vi "Get Custom Device Reference.vi"(8 "error in (no error)":errorcluster, 11 "Item Ref in":T1 format="%.0x") -> (0 "error out":errorcluster, 2 "Custom Device Ref":T1 format="%.0x", 3 "Item Ref out":T1 format="%.0x")   [LabVIEW 2020, in "Engine Simulation Toolkit System Explorer.lvlib"]
uses:
  Engine Simulation Toolkit System Explorer.lvlib
  <vilib>/NI VeriStand/Custom Device API/Custom Device Item Ref.ctl
  <vilib>/NI VeriStand/Custom Device Tools/Custom Device Utility Library/Search Direction.ctl
  Shared/Constants and GUIDs.vi
  <vilib>/NI VeriStand/Custom Device Tools/Custom Device Utility Library/NI VeriStand - Search for Item by GUID.vi
  <vilib>/NI VeriStand/Custom Device Tools/Custom Device Utility Library/Custom Device Utility Library.lvlib
  Shared/Engine Simulation Toolkit Shared.lvlib
  <vilib>/NI VeriStand/Custom Device API/Custom Device API.lvlib
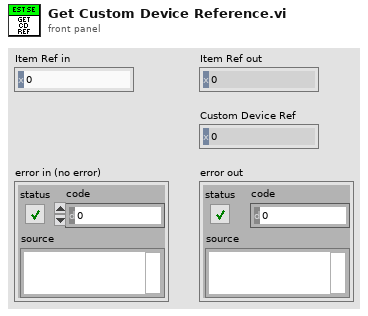
[diagram p1: front panel]
types:
  T1 = typedef "Custom Device API.lvlib/Custom Device Item Ref.ctl" = u64
  T2 = typedef "Custom Device Utility Library.lvlib/Search Direction.ctl" = enum16{"Down", "Up"}
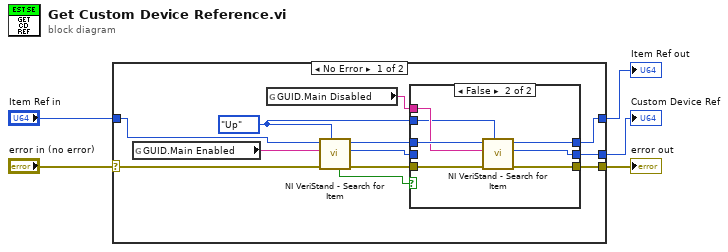
[diagram p0: block diagram]
diagram:
  n1 = case shown="No Error" "error in (no error)" {
    selector: "error in (no error)" -> [w6 w28]
    tunnel: [w17 w28] -> w5
    tunnel: [w16 _] -> w4
    tunnel: [w15 w29] -> w3
    tunnel: "Item Ref in" -> [w7 w29]
    frame No Error {
      w14 = Search_Direction."Up" ("Direction (Down)")
      n2 = global read "Constants and GUIDs.vi" "GUID.Main Enabled"() -> (w8:string)
      n3 = global read "Constants and GUIDs.vi" "GUID.Main Disabled"() -> (w13:string)
      n4 = call-poly <vilib>:"NI VeriStand - Search for Item.vi"("Direction (Down)"=w14, "error in"=w6, "Item GUID"=w8, "Section Ref in"=w7) -> ("error out"=w10:errorcluster, "Item Ref"=w12:T1, "Section Ref out"=w11:T1, "Found"=w9:bool)  [unwired: 4 in]
      n5 = case shown="False" w9 {
        tunnel: w10 -> [w20 w27]
        tunnel: w11 -> [w18 w26]
        tunnel: w12 -> [w19 _]
        tunnel: w13 -> [_ w25]
        tunnel: w14 -> [_ w24]
        tunnel: [w19 w23] -> w16
        tunnel: [w18 w22] -> w15
        tunnel: [w20 w21] -> w17
        frame True {
        }
        frame False {
          n6 = call-poly <vilib>:"NI VeriStand - Search for Item.vi"("Direction (Down)"=w24, "error in"=w27, "Item GUID"=w25, "Section Ref in"=w26) -> ("error out"=w21:errorcluster, "Item Ref"=w23:T1, "Section Ref out"=w22:T1)  [unwired: 4 in, 1 out]
        }
      }
    }
    frame Error {
    }
  }
  "error out" <- w5
  "Custom Device Ref" <- w4
  "Item Ref out" <- w3
